vi "ReadProfileName.vi"(8 "error in (no error)":errorcluster caption="错误输入（无错误）", 11 "ProfileNumber(from 0)":i32) -> (0 "error out":errorcluster caption="错误输出", 3 "Profile Names":string)   [LabVIEW 2010]
uses:
  NI Modbus.llb/MB Serial Master Query Read Input Registers (poly).vi
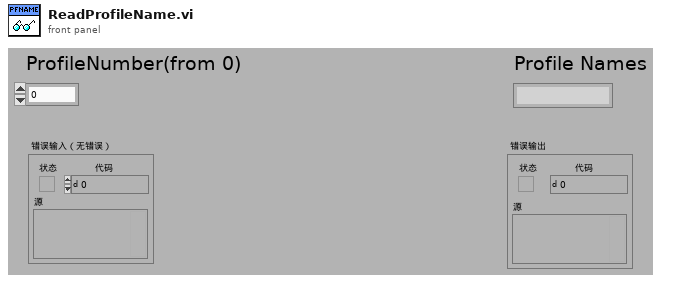
[diagram p1: front panel]
types:
  T1 = cluster{"Mode":enum16{"RTU", "ASCII"}, "Slave Address":u8}
  T2 = typedef "Path InitPaths__FS.ctl" = cluster{"Ctrller CFG":path, "INI":path, "Profile":path, "EventLog":path, "Data":path}
  T3 = typedef "Controller Configuration__CHC.ctl" = cluster{"Ctrller Type":T4, "Ctrller Name":string, "Ctrller Addr":string, "Server IP":string, "Conn Result":string, "Port":string, "Baud":dbl}
  T4 = typedef "Controller Configuration__Ctrller Type.ctl" = enum16{"F4S/D", "Synergy"}
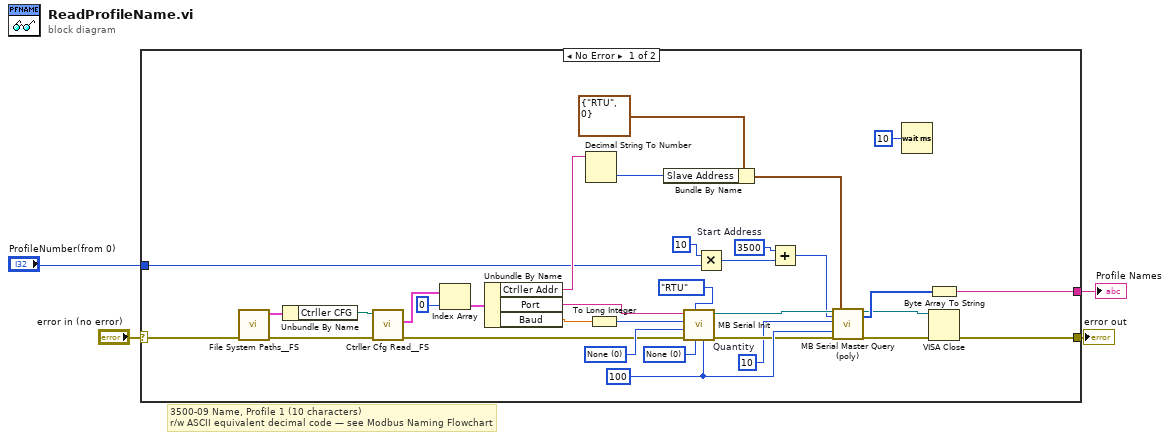
[diagram p0: block diagram]
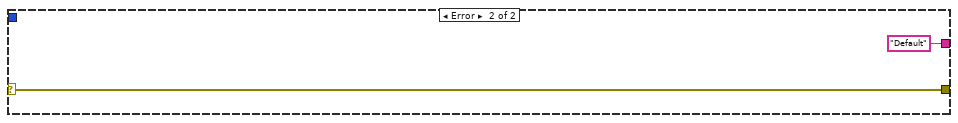
[diagram p2: hidden frame]
diagram:
  # "3500-09 Name, Profile 1 (10 characters)\nr/w ASCII equivalent decimal code — see Modbus Naming Flowchart"
  n1 = case shown="No Error" "error in (no error)" {
    selector: "error in (no error)" -> [w37 w39]
    tunnel: [w36 w39] -> w3
    tunnel: "ProfileNumber(from 0)" -> [w6 _]
    tunnel: [w5 "Default" ("string")] -> w1
    frame No Error {
      w12 = u16 10  # Quantity
      w32 = u32 100 ("Timeout")
      w31 = u16 0 items=["None", "XON/XOFF", "RTS/CTS", "XON/XOFF & RTS/CTS", "DTR/DSR", "XON/XOFF & DTR/DSR"] ("Flow Control")
      w29 = u16 0 items=["None", "Odd", "Even", "Mark", "Space"] ("Parity")
      w35 = 3500  # Start Address
      n2 = call "File System Paths__FS.vi"("error in (no error)"=w37) -> ("error out"=w20:errorcluster, "FilePaths"=w14:T2)  [unwired: 8 in, 1 out]
      n3 = Unbundle By Name(w14) -> ("Ctrller CFG"=w13:path)
      n4 = call "Ctrller Cfg Read__FS.vi"("error in (no error)"=w20, "Path In"=w13) -> ("error out"=w21:errorcluster, "Ctrllers"=w15:T3[])  [unwired: 7 in, 1 out]
      n5 = Index Array(array=w15, index=0) -> (element=w17:T3)
      n6 = Unbundle By Name(w17) -> ("Ctrller Addr"=w18:string, "Port"=w24:string, "Baud"=w19:dbl)
      n7 = Decimal String To Number(string=w18) -> (number=w28:i32)  [unwired: 2 in, 1 out]
      n8 = To Long Integer(number=w19) -> (32bit integer=w22:i32)
      n9 = Bundle By Name(cluster=T1 {"Mode"=enum."RTU", "Slave Address"=0} ("Serial Parameters"), "Slave Address"=w28) -> (w27:T1)
      n10 = call "MB Serial Init.vi"("Timeout"=w32, "Flow Control"=w31, "Mode"=enum16{"RTU", "ASCII"}."RTU", "error in (no error)"=w21, "Parity"=w29, "Baud Rate"=w22, "VISA resource name"=w24) -> ("error out"=w30:errorcluster, "VISA resource name out"=w25:refnum<visa-resource-name>)  [unwired: 3 in]
      n11 = Multiply(x=10, y=w6) -> (x*y=w33:i32)
      n12 = Add(x=w35, y=w33) -> (x+y=w11:i32)
      n13 = call-poly "MB Serial Master Query (poly).vi"("VISA resource name"=w25, "Starting Address"=w11, "Quantity"=w12, "Timeout"=w32, "error in"=w30, "Serial Parameters"=w27) -> ("VISA resource name out"=w9:refnum<visa-resource-name>, "Input Registers"=w10:u16[], "error out"=w8:errorcluster)  [unwired: 10 in, 1 out]
      n14 = Wait (ms)(milliseconds to wait=u32 10) -> ()  [unwired: 1 out]
      n15 = Byte Array To String(unsigned byte array=w10) -> (string=w5:string)
      n16 = VISA Close(VISA resource name=w9, error in (no error)=w8) -> (error out=w36:errorcluster)
    }
    frame Error {
    }
  }
  "error out" <- w3
  "Profile Names" <- w1
